vi "Read Scale.vi"(8 "error in (no error)":errorcluster, 11 "O3 Frequency Train Actor in":refnum<class "O3 Frequency Train Actor.lvclass">) -> (0 "error out":errorcluster, 2 "Scale":dbl, 3 "O3 Frequency Train Actor out":refnum<class "O3 Frequency Train Actor.lvclass">)   [LabVIEW 2014, in "Calibration.lvlib" / "O3 Frequency Train Actor.lvclass"]
uses:
  O3 Frequency Train Actor.lvclass
  O3 Frequency Train Actor.lvclass/O3 Frequency Train Actor.ctl
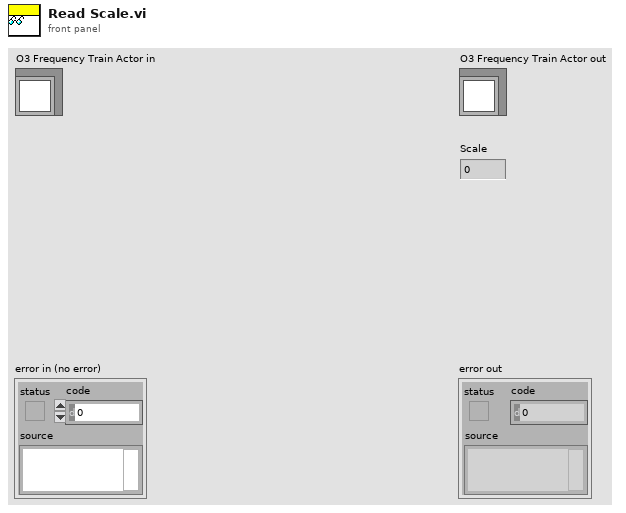
[diagram p1: front panel]
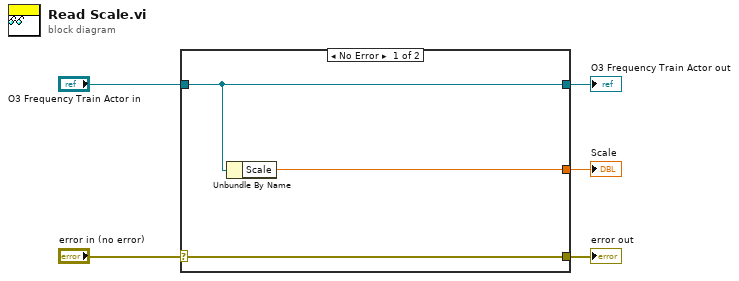
[diagram p0: block diagram]
diagram:
  n1 = case shown="No Error" "error in (no error)" {
    selector: "error in (no error)" -> [w8 w9]
    tunnel: [w8 w9] -> w4
    tunnel: [w7 w10] -> w2
    tunnel: "O3 Frequency Train Actor in" -> [w7 w10]
    tunnel: [w6 _] -> w1
    frame No Error {
      n2 = Unbundle By Name(w7) -> ("Scale"=w6:dbl)
    }
    frame Error {
    }
  }
  "error out" <- w4
  "O3 Frequency Train Actor out" <- w2
  "Scale" <- w1
